vi "niDTS BT INSTR TX Configure BT Basic Parameters.vi"(8 "error in (no error)":errorcluster, 11 "niDTS BT INSTR TX in":refnum<class "niDTS BT INSTR TX.lvclass">) -> (0 "error out":errorcluster, 3 "niDTS BT INSTR TX out":refnum<class "niDTS BT INSTR TX.lvclass">)   [LabVIEW 2015, in "niDTS BT.lvlib" / "niDTS BT INSTR TX.lvclass"]
uses:
  niDTS BT INSTR TX.lvclass
  niDTS BT INSTR TX.lvclass/niDTS BT INSTR TX.ctl
  RiviInstDriver/niRfsaBT/Objects/niRfsaBt.lvclass
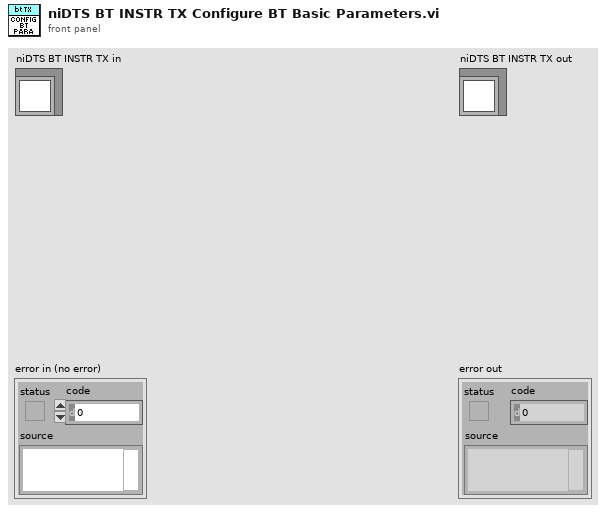
[diagram p1: front panel]
types:
  T1 = typedef "niRfsaBT.lvclass/niRfsaBT INC Handle.ctl" = refnum<data-value>
  T2 = typedef "niDTS BT.lvlib/niDTS BT INC Packet Type.ctl" = enum16{"NULL", "POLL", "FHS", "DM1", "DH1", "HV1", "HV2", "HV3", "EV3", "DV", "AUX1", "DM3", "DH3", "EV4", "EV5", "DM5", "DH5", "LE-TP"}
  T3 = cluster{"PacketType":enum16{"DH1", "DH3", "DH5", "LETP"}, "PacketPayloadDatarate":i32}
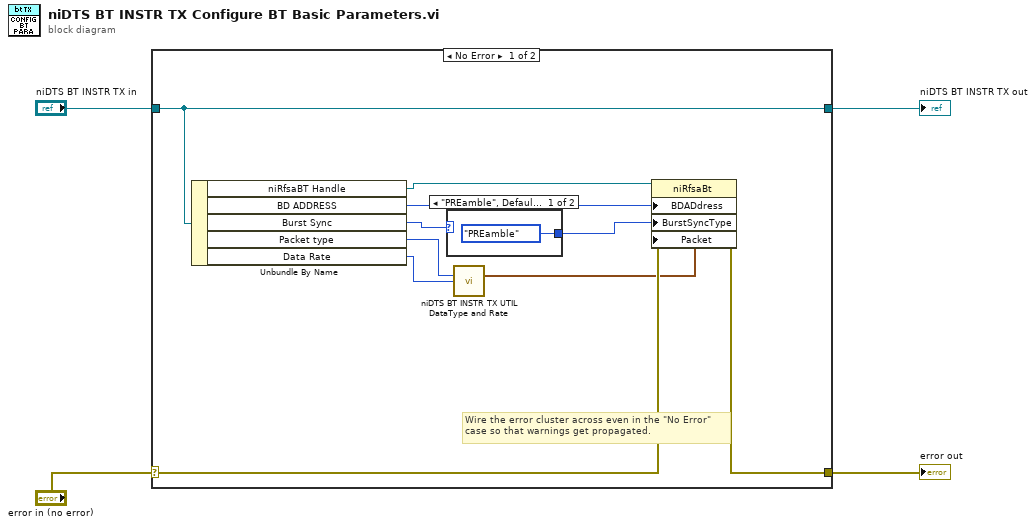
[diagram p0: block diagram]
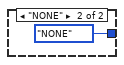
[diagram p2: hidden frame]
diagram:
  n1 = case shown="No Error" "error in (no error)" {
    selector: "error in (no error)" -> [w13 w18]
    tunnel: [w12 w18] -> w3
    tunnel: [w14 w17] -> w1
    tunnel: "niDTS BT INSTR TX in" -> [w14 w17]
    frame No Error {
      # "Wire the error cluster across even in the \"No Error\"\ncase so that warnings get propagated."
      n2 = Unbundle By Name(w14) -> ("niRfsaBT Handle"=w10:T1, "BD ADDRESS"=w11:u32, "Burst Sync"=w8:enum16{"NONE", "PREamble"}, "Packet type"=w7:T2, "Data Rate"=w6:i32)
      n3 = case shown="\"PREamble\", Default" w8 {
        tunnel: [enum16{"PREamble", "NONE"}."PREamble" ("CONFigure:RFSA:BLUetooth:BurstSyncType") enum16{"PREamble", "NONE"}."NONE" ("CONFigure:RFSA:BLUetooth:BurstSyncType")] -> w5
        frame "PREamble", Default {
        }
        frame "NONE" {
        }
      }
      n4 = call "niDTS BT INSTR TX UTIL DataType and Rate.vi"("Packet type"=w7, "Data Rate"=w6) -> ("Packet"=w9:T3)  [unwired: 13 in]
      n5 = property class="niRfsaBt"(reference=w10, error in=w13, "BDADdress"=w11, "BurstSyncType"=w5, "Packet"=w9) -> (error out=w12:errorcluster)  [unwired: 1 out]
    }
    frame Error {
    }
  }
  "error out" <- w3
  "niDTS BT INSTR TX out" <- w1
